vi "Authenticate.vi"(8 "error in (no error)":errorcluster, 10 "Authentication Inputs":T2, 11 "FormAuthentication in":refnum<class "FormAuthentication.lvclass">) -> (0 "error out":errorcluster, 2 "Authentication Outputs":T1, 3 "FormAuthentication out":refnum<class "FormAuthentication.lvclass">)   [LabVIEW 2020, in "HTTP Server.lvlib" / "FormAuthentication.lvclass"]
uses:
  FormAuthentication.lvclass
  Authentication Inputs.ctl
  Session/Session.lvclass
  <vilib>/IlluminatedG/IG HTTP Utils/HTTP Utils/Request/Request.lvclass
  User Provider/User Provider.lvclass
  Password Encoder/Password Encoder.lvclass
  Authentication Outputs.ctl
  User/User.lvclass
  FormAuthentication.lvclass/FormAuthentication.ctl
  HTTP Server.lvlib
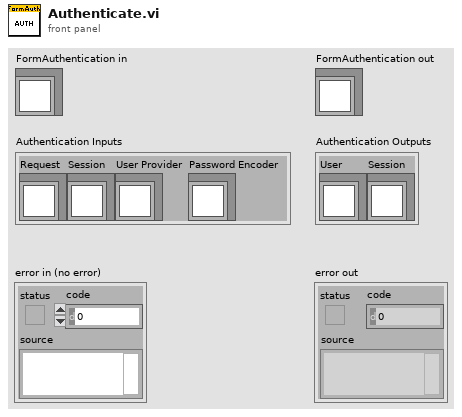
[diagram p1: front panel]
types:
  T1 = typedef "HTTP Server.lvlib/Authentication Outputs.ctl" = cluster{"User":refnum<class "User.lvclass">, "Session":refnum<class "Session.lvclass">}
  T2 = typedef "HTTP Server.lvlib/Authentication Inputs.ctl" = cluster{"Request":refnum<class "Request.lvclass">, "Session":refnum<class "Session.lvclass">, "User Provider":refnum<class "User Provider.lvclass">, "Password Encoder":refnum<class "Password Encoder.lvclass">}
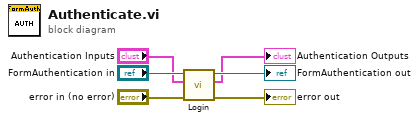
[diagram p0: block diagram]
diagram:
  n1 = call "Login.vi"("error in (no error)"="error in (no error)", "Authentication Inputs"="Authentication Inputs", "FormAuthentication in"="FormAuthentication in") -> ("error out"=→"error out":errorcluster, "Authentication Outputs"=→"Authentication Outputs":T1, "FormAuthentication out"=→"FormAuthentication out":refnum<class "FormAuthentication.lvclass">)  [unwired: 6 in]
